vi "add_control.vi"(7 "Add Control Type":T5, 8 "error in (no error)":errorcluster, 9 "Single Control Spec":T1, 10 "BD Position":cluster{"Left":i32, "Top":i32}={"Left"=75, "Top"=60}, 11 "VI Ref In":refnum<vi>) -> (0 "error out":errorcluster, 2 "Control Ref Out":refnum<vi>, 3 "VI Ref Out":refnum<vi>)   [LabVIEW 2018]
uses:
  TypeDefinitions/bd_control_type.ctl
  TypeDefinitions/single_control_spec.ctl
  TypeDefinitions/control_data_type.ctl
  TypeDefinitions/control_class.ctl
  TypeDefinitions/ring_string_and_value.ctl
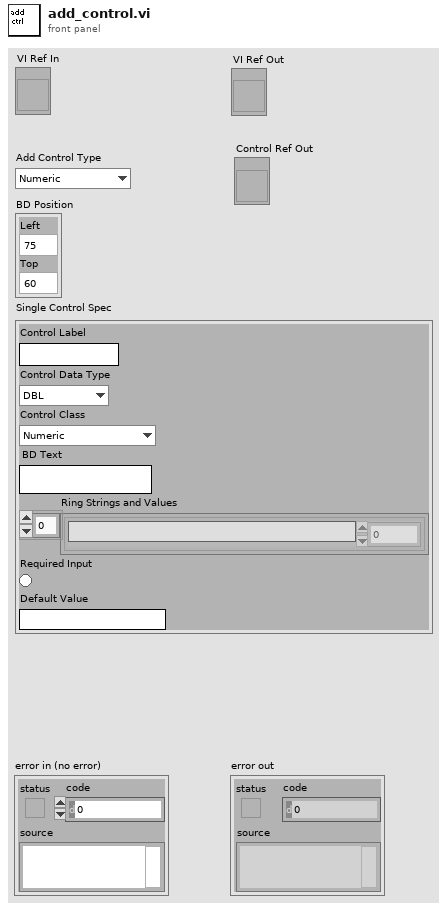
[diagram p1: front panel]
types:
  T1 = typedef "single_control_spec.ctl" = cluster{"Control Label":string, "Control Data Type":T2, "Control Class":T3, "BD Text":string, "Ring Strings and Values":T4[], "Required Input":bool, "Default Value":string}
  T2 = typedef "control_data_type.ctl" = enum16{"DBL", "I32", "Boolean", "String", "U16", "U32", "EXT", "SGL", "I16", "U8", "I8", "I64", "U64", "Waveform", "Reference", "Variant", "Cluster"}
  T3 = typedef "control_class.ctl" = enum16{"Numeric", "Vertical Slide Switch", "Text Ring", "String", "Array", "VISAName", "WaveformGraph", "Cluster"}
  T4 = typedef "ring_string_and_value.ctl" = cluster{"String":string, "Value":dbl}
  T5 = typedef "bd_control_type.ctl" = enum16{"Numeric", "Ring", "Boolean", "String", "VisaIn", "VisaOut", "Error In", "Error Out", "Array", "Waveform"}
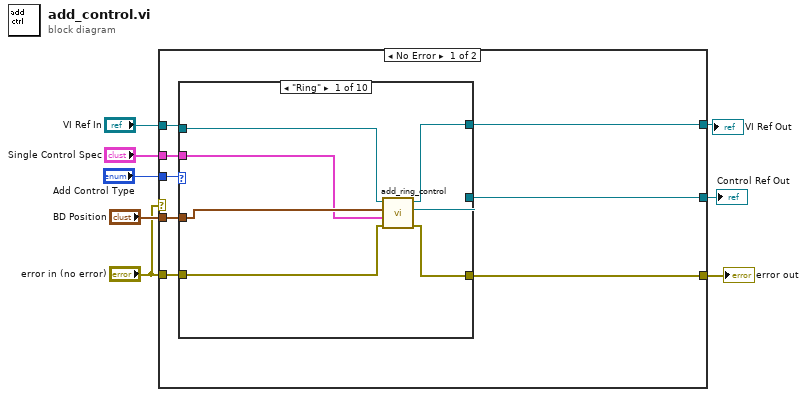
[diagram p0: block diagram]
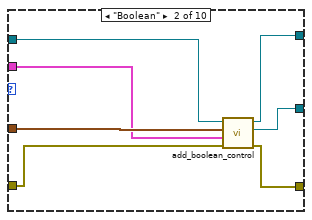
[diagram p2: hidden frame]
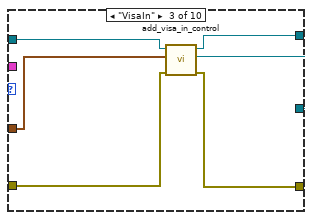
[diagram p3: hidden frame]
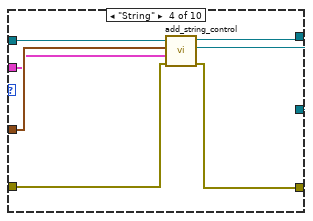
[diagram p4: hidden frame]
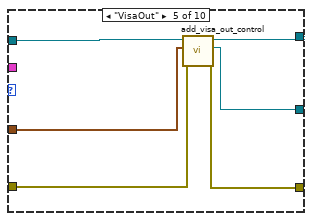
[diagram p5: hidden frame]
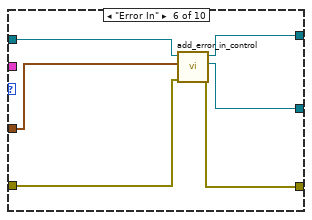
[diagram p6: hidden frame]
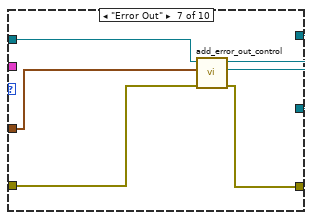
[diagram p7: hidden frame]
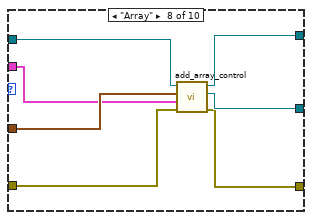
[diagram p8: hidden frame]
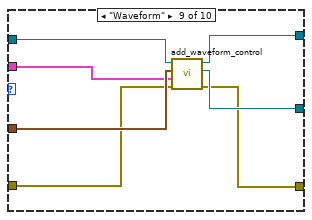
[diagram p9: hidden frame]
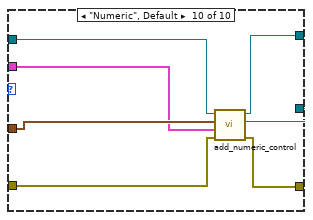
[diagram p10: hidden frame]
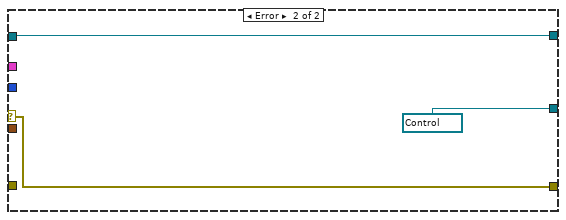
[diagram p11: hidden frame]
diagram:
  n1 = case shown="No Error" "error in (no error)" {
    selector: "error in (no error)" -> [_ w85]
    tunnel: "Add Control Type" -> [w16 _]
    tunnel: [w9 w85] -> w7
    tunnel: "error in (no error)" -> [w15 _]
    tunnel: "VI Ref In" -> [w14 w84]
    tunnel: [w13 w84] -> w5
    tunnel: "BD Position" -> [w12 _]
    tunnel: "Single Control Spec" -> [w11 _]
    tunnel: [w10 refnum<vi> refnum ("Control Ref Out")] -> w1
    frame No Error {
      n2 = case shown="\"Ring\"" w16 {
        tunnel: w14 -> [w23 w30 w36 w43 w47 w55 w61 w68 w72 w82]
        tunnel: [w22 w29 w32 w38 w49 w54 w57 w67 w73 w81] -> w13
        tunnel: [w21 w28 w33 w39 w48 w53 w58 w63 w74 w78] -> w9
        tunnel: w15 -> [w20 w27 w34 w40 w45 w52 w59 w62 w69 w79]
        tunnel: w12 -> [w19 w26 w35 w42 w46 w51 w60 w66 w71 w80]
        tunnel: w11 -> [w18 w25 _ w41 _ _ _ w65 w70 w77]
        tunnel: [w17 w24 w31 w37 w44 w50 w56 w64 w75 w76] -> w10
        frame "Ring" {
          n3 = call "add_ring_control.vi"("error in (no error)"=w20, "Single Control Spec"=w18, "BD Position"=w19, "VI Ref In"=w23) -> ("error out"=w21:errorcluster, "Control Ref Out"=w17:refnum<vi>, "VI Ref Out"=w22:refnum<vi>)  [unwired: 1 in, 4 out]
        }
        frame "Boolean" {
          n4 = call "add_boolean_control.vi"("error in (no error)"=w27, "Single Control Spec"=w25, "BD Position"=w26, "VI Ref In"=w30) -> ("error out"=w28:errorcluster, "Control Ref Out"=w24:refnum<vi>, "VI Ref Out"=w29:refnum<vi>)  [unwired: 1 in, 4 out]
        }
        frame "VisaIn" {
          n5 = call "add_visa_in_control.vi"("error in (no error)"=w34, "BD Position"=w35, "VI Ref In"=w36) -> ("error out"=w33:errorcluster, "Control Ref Out"=w31:refnum<vi>, "VI Ref Out"=w32:refnum<vi>)  [unwired: 6 out]
        }
        frame "String" {
          n6 = call "add_string_control.vi"("error in (no error)"=w40, "Single Control Spec"=w41, "BD Position"=w42, "VI Ref In"=w43) -> ("error out"=w39:errorcluster, "Control Ref Out"=w37:refnum<vi>, "VI Ref Out"=w38:refnum<vi>)  [unwired: 5 out]
        }
        frame "VisaOut" {
          n7 = call "add_visa_out_control.vi"("error in (no error)"=w45, "BD Position"=w46, "VI Ref In"=w47) -> ("error out"=w48:errorcluster, "Control Ref Out"=w44:refnum<vi>, "VI Ref Out"=w49:refnum<vi>)  [unwired: 6 out]
        }
        frame "Error In" {
          n8 = call "add_error_in_control.vi"("error in (no error)"=w52, "BD Position"=w51, "VI Ref In"=w55) -> ("error out"=w53:errorcluster, "Control Ref Out"=w50:refnum<vi>, "VI Ref Out"=w54:refnum<vi>)  [unwired: 6 out]
        }
        frame "Error Out" {
          n9 = call "add_error_out_control.vi"("error in (no error)"=w59, "BD Position"=w60, "VI Ref In"=w61) -> ("error out"=w58:errorcluster, "Control Ref Out"=w56:refnum<vi>, "VI Ref Out"=w57:refnum<vi>)  [unwired: 6 out]
        }
        frame "Array" {
          n10 = call "add_array_control.vi"("error in (no error)"=w62, "Single Control Spec"=w65, "BD Position"=w66, "VI Ref In"=w68) -> ("error out"=w63:errorcluster, "Arr Refnum"=w64:refnum<vi>, "VI Ref Out"=w67:refnum<vi>)  [unwired: 1 in, 4 out]
        }
        frame "Waveform" {
          n11 = call "add_waveform_control.vi"("error in (no error)"=w69, "Single Control Spec"=w70, "BD Position"=w71, "VI Ref In"=w72) -> ("error out"=w74:errorcluster, "WFGraph Refnum"=w75:refnum<vi>, "VI Ref Out"=w73:refnum<vi>)  [unwired: 5 out]
        }
        frame "Numeric", Default {
          n12 = call "add_numeric_control.vi"("error in (no error)"=w79, "Single Control Spec"=w77, "BD Position"=w80, "VI Ref In"=w82) -> ("error out"=w78:errorcluster, "Control Ref Out"=w76:refnum<vi>, "VI Ref Out"=w81:refnum<vi>)  [unwired: 1 in, 4 out]
        }
      }
    }
    frame Error {
    }
  }
  "error out" <- w7
  "VI Ref Out" <- w5
  "Control Ref Out" <- w1
